vi "bulk write.vi"(7 "timeout":i32, 9 "size":i32, 10 "element":i8, 11 "ep":i32) -> (3 "len":i32)   [LabVIEW 2013, in "libusvlv.lvlib"]
doc: "extern \"C\" int _declspec_dll_use bulk_write(int ep, char* bytes, int size, int timeout);"
uses:
  libusvlv.lvlib
  UsbCom.dll
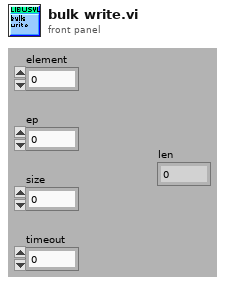
[diagram p1: front panel]
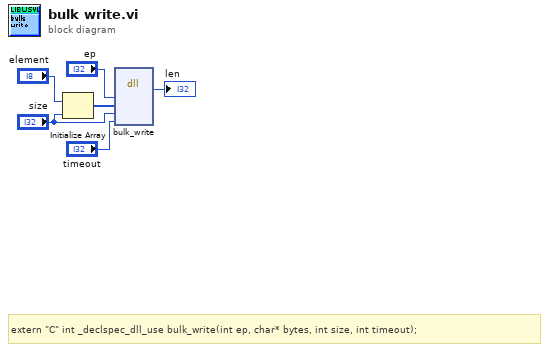
[diagram p0: block diagram]
diagram:
  # "extern \"C\" int _declspec_dll_use bulk_write(int ep, char* bytes, int size, int timeout);"
  n1 = Initialize Array("element", "size") -> (w1:i8[])
  n2 = dll-call lib="E:/libusvlv/UsbCom.dll" fn="bulk_write"("ep"="ep", "bytes"=w1, "size"="size", "timeout"="timeout") -> ("返回类型"=→"len":i32)  [unwired: 7 in, 2 out]
